vi "stm_GetIDfromName_.vi"(9 "Name":string, 11 "MetaData":T1[](array[typedef])) -> (1 "Found":bool, 3 "Meta ID":u16)   [LabVIEW 2010]
doc: "This VI looks up the Meta data index using the Meta data name.\n\nCopyright 2015, 2016, 2017 National Instruments Corporation\n\nLicensed under the Apache License, Version 2.0 (the \"License\"); you may not use this file except in compliance with the License.\n\n You may obtain a copy of the License at\n\n http://www.apache.org/licenses/LICENSE-2.0\n\nUnless required by applicable law or agreed to in writing, software distributed under the License is distributed on an \"AS IS\" BASIS, WITHOUT WARRANTIES OR CONDITIONS OF ANY KIND, either express or implied.\n\nSee the License for the specific language governing permissions and limitations under the License."
uses:
  stm_MetaDataElement.ctl
  NI STM.lvlib
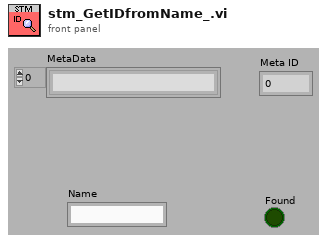
[diagram p1: front panel]
types:
  T1 = typedef "stm_MetaDataElement.ctl" = string
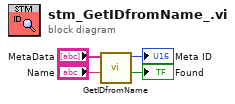
[diagram p0: block diagram]
diagram:
  n1 = call "GetIDfromName.vi"("name"="Name", "meta data"="MetaData") -> ("found?"=→"Found":bool, "meta ID"=→"Meta ID":u16)  [unwired: 8 in]
